vi "IMAQ FPGA Configure Image Transfer from Target.vi"   [LabVIEW 2020, in "NI_VDM_FPGA_Basics.lvlib"]
doc: "Configures the transfer of an image from the target FPGA to the host processor via a DMA FIFO. If the <B>Image Size</B> control specifies non-zero <B>Width</B> and <B>Height</B> values, then the image referenced by Image will be resized to match those values. Otherwise, the original image size is preserved. In addition, a reference will be opened to the DMA FIFO that will be used to transfer the image from the target FPGA to the host computer."
uses:
  <vilib>/visionFPGA/NI_VDM_FPGA_Basics.lvlib
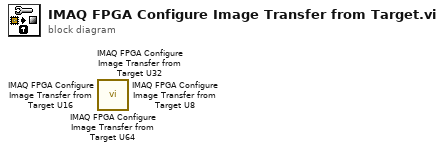
[diagram p0: block diagram]
diagram:
  n1 = call <vilib>:"IMAQ FPGA Configure Image Transfer from Target U64.vi"() -> ()  [unwired: 9 in, 3 out]
  n2 = call <vilib>:"IMAQ FPGA Configure Image Transfer from Target U32.vi"() -> ()  [unwired: 9 in, 3 out]
  n3 = call <vilib>:"IMAQ FPGA Configure Image Transfer from Target U16.vi"() -> ()  [unwired: 9 in, 3 out]
  n4 = call <vilib>:"IMAQ FPGA Configure Image Transfer from Target U8.vi"() -> ()  [unwired: 9 in, 3 out]
